vi "5646R Coherency Test View Data.vi"() -> ()   [LabVIEW 2019]
doc: "Use this example to learn the basics of TClk synchronization for RF vector signal analyzers and generators. This example shows how to create NI-RFSA and NI-RFSG sessions and pass them to NI-TClk synchronization functions. It uses NI-TClk to make the NI-RFSA and NI-RFSG start at the same time."
uses:
  <instrlib>/niRFSA/niRFSA.llb/niRFSA Get IQ Components (Complex Cluster).vi
panel:
  in  "RX Sample Rate: 1MSps 2":cluster{"t0":dbl, "dt":dbl, "Y":cdb[]}={"t0"=0.0, "dt"=9.99999999998778e-07, "Y"=array[20000 elements]} caption="RX Sample Rate: 1MSps" {"Y" format="%_2g"; "dt" format="%.6p"; "t0" format="%.6p"}
  in  "RX Sample Rate: 100KSps":cluster{"t0":dbl, "dt":dbl, "Y":cdb[]}={"t0"=0.0, "dt"=9.99999999984567e-06, "Y"=array[20000 elements]} {"Y" format="%_2g"; "dt" format="%.6p"; "t0" format="%.6p"}
  in  "RX Sample Rate: 1MSps":cluster{"t0":dbl, "dt":dbl, "Y":cdb[]}={"t0"=0.0, "dt"=9.99999999998778e-07, "Y"=array[20000 elements]} {"Y" format="%_2g"; "dt" format="%.6p"; "t0" format="%.6p"}
  in  "RX Sample Rate: 10MSps":cluster{"t0":dbl, "dt":dbl, "Y":cdb[]}={"t0"=0.0, "dt"=9.999999999998438e-08, "Y"=array[20000 elements]} {"Y" format="%_2g"; "dt" format="%.6p"; "t0" format="%.6p"}
  in  "RX Sample Rate: 100MSps":cluster{"t0":dbl, "dt":dbl, "Y":cdb[]}={"t0"=0.0, "dt"=9.999999999999858e-09, "Y"=array[20000 elements]} {"Y" format="%_2g"; "dt" format="%.6p"; "t0" format="%.6p"}
  in  "RX Sample Rate: 100KSps":cluster{"t0":dbl, "dt":dbl, "Y":cdb[]}={"t0"=0.0, "dt"=9.99999999984567e-06, "Y"=array[20000 elements]} {"Y" format="%_2g"; "dt" format="%.6p"; "t0" format="%.6p"}
  out "error out":errorcluster {"code" format="%.0x"}
  in  "Remove Frequency Offset":bool
  out "Amplitude Stability":dbl format="%.6p"
  out "Phase Stability":dbl format="%.6p"
  in  "Tab Control":enum32{"     IQ Data", "Magnitude", "Phase"}(tab)
  out "IQ Data":cluster{"t0":dbl, "dt":dbl, "Y":dbl[]}[](graph)
  out "Magnitude":cluster{"t0":dbl, "dt":dbl, "Y":dbl[]}(graph)
  out "Phase":cluster{"t0":dbl, "dt":dbl, "Y":dbl[]}(graph)
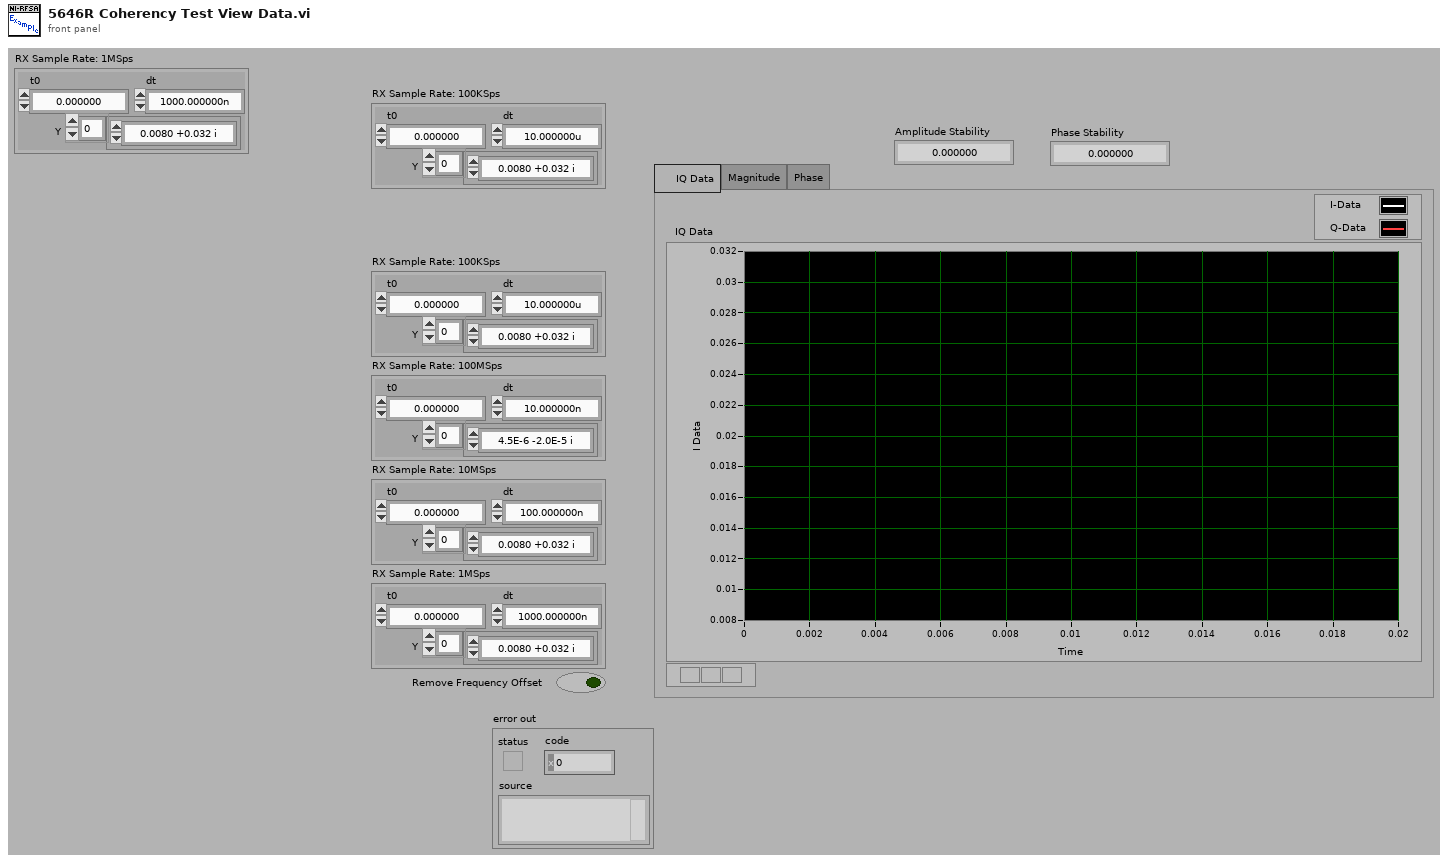
[diagram p1: front panel]
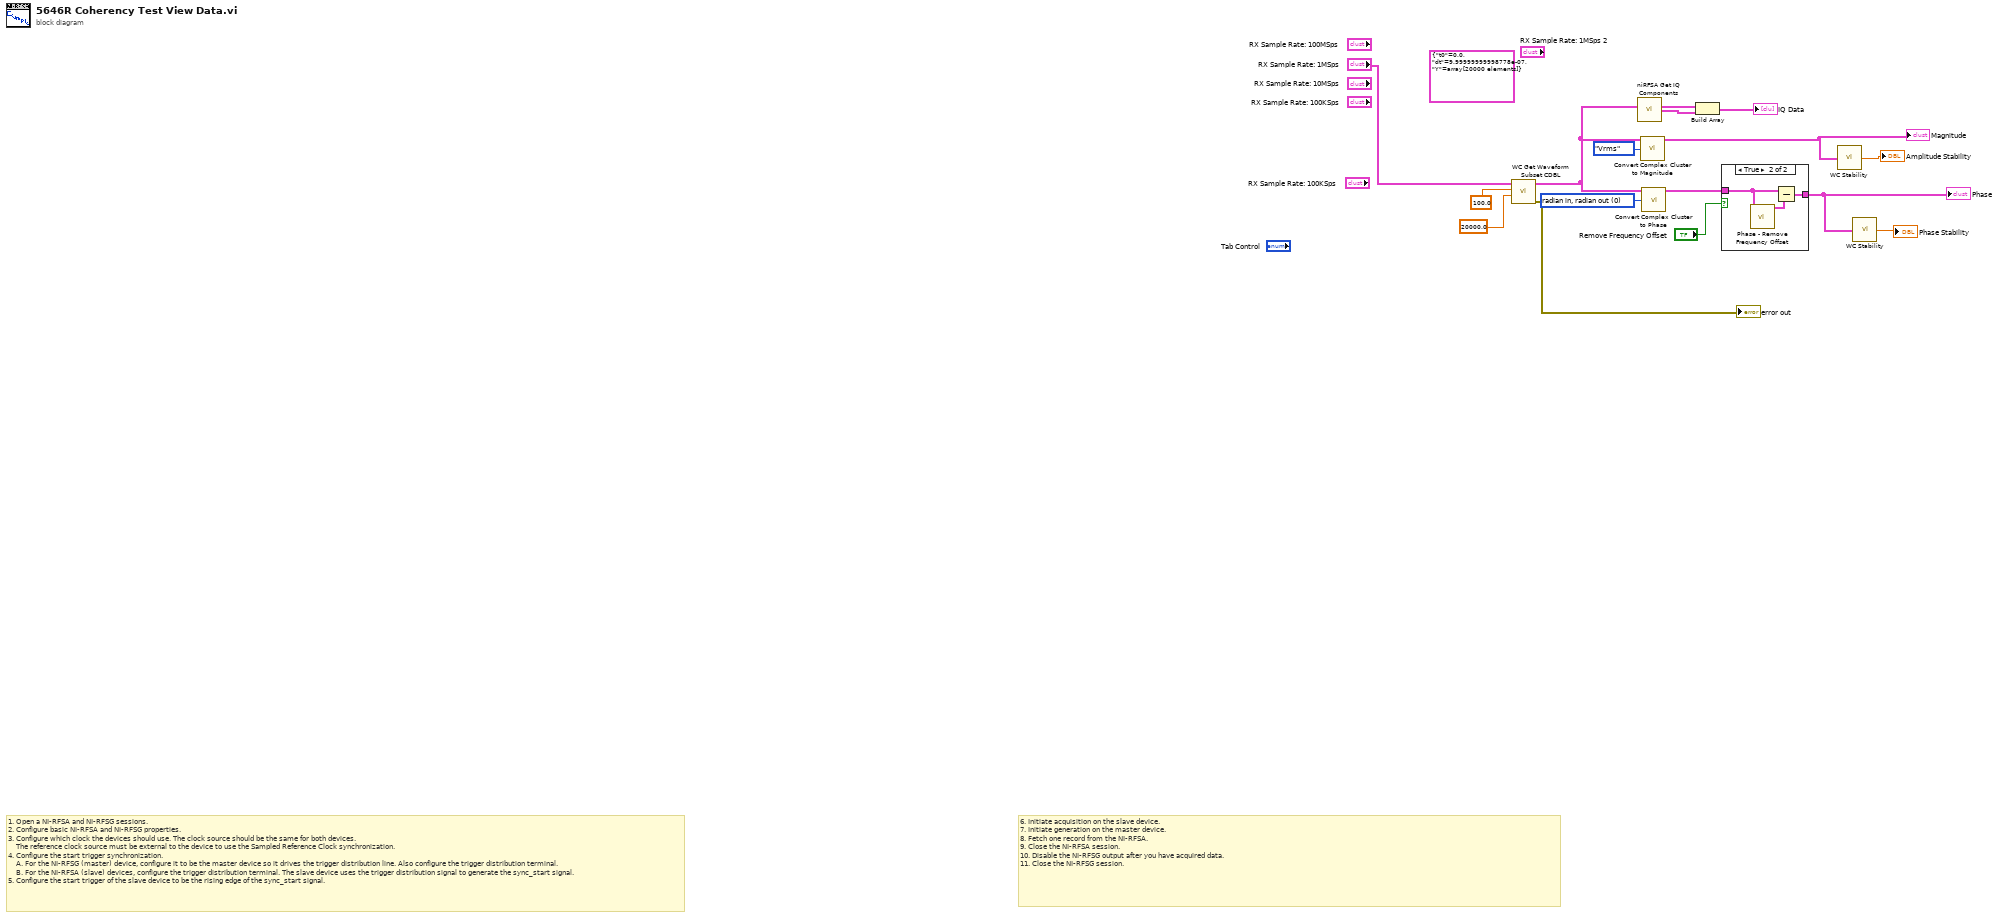
[diagram p0: block diagram]
diagram:
  (unwired) cluster{"t0":dbl, "dt":dbl, "Y":cdb[]} {"t0"=0.0, "dt"=9.99999999998778e-07, "Y"=array[20000 elements]} ("RX Sample Rate: 1MSps 2")
  w15 = 0 items=["radian in, radian out", "radian in, degree out", "degree in, degree out", "degree in, radian out"] ("phase unit")
  # "6. Initiate acquisition on the slave device.\n7. Initiate generation on the master device.\n8. Fetch one record from the NI-RFSA.\n9. Close the NI-RFSA session.\n10. Disable the NI-RFSG output after you have acquired data.\n11. Close the NI-RFSG session."
  # "1. Open a NI-RFSA and NI-RFSG sessions.\n2. Configure basic NI-RFSA and NI-RFSG properties.\n3. Configure which clock the devices should use. The clock source should be the same for both devices.\n    The reference clock source must be external to the device to use the Sampled Reference Clock synchronization.\n4. Configure the start trigger synchronization.\n    A. For the NI-RFSG (master) device, configure it to be the master device so it drives the trigger distribution line. Also configure the trigger distribution terminal.\n    B. For the NI-RFSA (slave) devices, configure the trigger distribution terminal. The slave device uses the trigger distribution signal to generate the sync_start signal.\n5. Configure the start trigger of the slave device to be the rising edge of the sync_start signal."
  n1 = call "WC Get Waveform Subset CDBL.vi"("duration"=20000.0, "start samples/time"=100.0, "Waveform In"="RX Sample Rate: 1MSps") -> ("error out"=→"error out":errorcluster, "Waveform Out"=w12:cluster{"t0":dbl, "dt":dbl, "Y":cdb[]})  [unwired: 3 in, 2 out]
  n2 = call-poly <instrlib>:"niRFSA Get IQ Components.vi"("data"=w12) -> ("I"=w14:cluster{"t0":dbl, "dt":dbl, "Y":dbl[]}, "Q"=w13:cluster{"t0":dbl, "dt":dbl, "Y":dbl[]})  [unwired: 1 in, 12 out]
  n3 = call "Convert Complex Cluster to Magnitude.vi"("IQ data (complex) In"=w12, "Public.Units"=enum8{"Vrms", "dBm"}."Vrms") -> ("Magnitude Out"=w4:cluster{"t0":dbl, "dt":dbl, "Y":dbl[]})  [unwired: 12 in, 1 out]
  "Magnitude" <- w4
  n4 = call "Convert Complex Cluster to Phase.vi"("IQ data (complex) In"=w12, "phase unit"=w15) -> ("Phase Out"=w11:cluster{"t0":dbl, "dt":dbl, "Y":dbl[]})  [unwired: 12 in, 1 out]
  n5 = Build Array(w14, w13) -> (→"IQ Data":cluster{"t0":dbl, "dt":dbl, "Y":dbl[]}[])
  n6 = case shown="True" "Remove Frequency Offset" {
    tunnel: w11 -> [w17 w19]
    tunnel: [w17 w18] -> w3
    frame False {
    }
    frame True {
      n7 = call "Phase - Remove Frequency Offset.vi"("Phase In"=w19) -> ("Phase Out"=w20:cluster{"t0":dbl, "dt":dbl, "Y":dbl[]})  [unwired: 13 in, 1 out]
      n8 = Subtract(x=w19, y=w20) -> (x-y=w18:cluster{"t0":dbl, "dt":dbl, "Y":dbl[]})
    }
  }
  "Phase" <- w3
  n9 = call "WC Stability.vi"("Data In"=w4) -> ("Stability"=→"Amplitude Stability":dbl)  [unwired: 4 in]
  n10 = call "WC Stability.vi"("Data In"=w3) -> ("Stability"=→"Phase Stability":dbl)  [unwired: 4 in]
